vi "Transfer Max Bin Amplitudes.vi"   [LabVIEW 2014]
doc: "This subVI performs the communication with the microcontroller through DMA. FPGA sends informations about FFT amplitudes and bin."
uses:
  <vilib>/rvi/Emulation/niFpgaEmulationIsFPGAContextNoSignature.vi
  <vilib>/rvi/DataTransferAndStorage/Container/Common/niFpgaContainerGetUniqueNameForEmu.vi
  <vilib>/rvi/Memory/Memory_Emulation/niFpgaMemoryEmulationCacheClearOnFirstRun.vi
  <vilib>/rvi/Memory/Memory_Emulation/nirvimemoryEmulationManagerCache_MakeExclusive.vi
  <vilib>/rvi/Memory/Memory_Emulation/niFpgaMemoryEmulationValidateCache.vi
  <vilib>/rvi/Memory/Memory_Emulation/nirvimemoryEmulationManagerCache_InsertValue.vi
  <vilib>/Utility/error.llb/Clear Errors.vi
  <vilib>/rvi/Memory/Memory_Emulation/nirvimemoryEmulationManagerCache_ReleaseExclusive.vi
  <vilib>/rvi/Memory/Memory_Emulation/nirvimemoryEmulationManagerCache_GetValue.vi
  <vilib>/rvi/Memory/Memory_Emulation/nirvimemoryEmulationManagerCache_SetValue.vi
  <vilib>/rvi/Emulation/niFpgaProcessEmulError.vi
  <vilib>/rvi/Emulation/niFpgaSctlEmulationGetInTimedLoop.vi
  <vilib>/rvi/interface/RandomDataEmulation/niFpgaRandomDataHandleErrors.vi
  <vilib>/rvi/DataTransferAndStorage/Container/XNode/niFpgaContainer.xnode
  <vilib>/rvi/DataTransferAndStorage/Register/Emulation/niFpgaRegisterEmulation.vi
  <vilib>/rvi/interface/RandomDataEmulation/nirviRandomDataFpgaReadWriteTemplate.vi
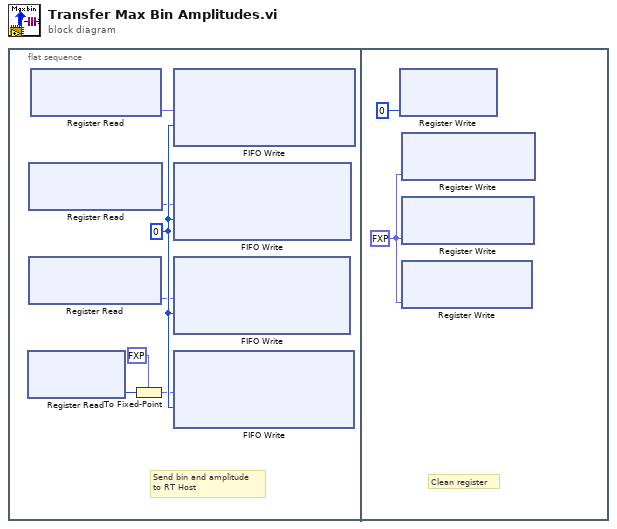
[diagram p0: block diagram]
diagram:
  n1 = flat-sequence {
    frame #0 {
      w7 = 0 ("Timeout")
      # "Send bin and amplitude\nto RT Host"
      n2 = xnode ("Register Read")() -> ("Data"=w3:i32)  [unwired: 1 in, 1 out]
      n3 = xnode ("Register Read")() -> ("Data"=w5:fxp<+,44,44>)  [unwired: 1 in, 1 out]
      n4 = xnode ("Register Read")() -> ("Data"=w4:fxp<+,44,44>)  [unwired: 1 in, 1 out]
      n5 = xnode ("Register Read")() -> ("Data"=w6:fxp<+,44,44>)  [unwired: 1 in, 1 out]
      n6 = To Fixed-Point(fixed-point type=fxp<+/-,12,12> 0.0 ("Element"), number=w3) -> (fixed-point=w1:fxp<+/-,12,12>)
      n7 = xnode ("FIFO Write")("Element"=w6, "Timeout"=w7) -> ()  [unwired: 1 in, 2 out]
      n8 = xnode ("FIFO Write")("Element"=w5, "Timeout"=w7) -> ()  [unwired: 1 in, 2 out]
      n9 = xnode ("FIFO Write")("Element"=w4, "Timeout"=w7) -> ()  [unwired: 1 in, 2 out]
      n10 = xnode ("FIFO Write")("Element"=w1, "Timeout"=w7) -> ()  [unwired: 1 in, 2 out]
    }
    frame #1 {
      w8 = fxp<+,44,44> 0.0 ("Data")
      # "Clean register"
      n11 = xnode ("Register Write")("Data"=0) -> ()  [unwired: 1 in, 1 out]
      n12 = xnode ("Register Write")("Data"=w8) -> ()  [unwired: 1 in, 1 out]
      n13 = xnode ("Register Write")("Data"=w8) -> ()  [unwired: 1 in, 1 out]
      n14 = xnode ("Register Write")("Data"=w8) -> ()  [unwired: 1 in, 1 out]
    }
  }
